vi "LESSON2_VIDEO8_CREATING_FIRST_APPLICATION.vi"() -> ()   [LabVIEW 2022 SP3]
panel:
  in  "Stop Button":bool
  out "Temperature Chart":dbl(graph)
  in  "Delay Multiplier":dbl(knob) scale=0.0..1.0
  in  "Number of Measurements":dbl
  # "This front panel shows chart numeric control and delay multiplier knob"
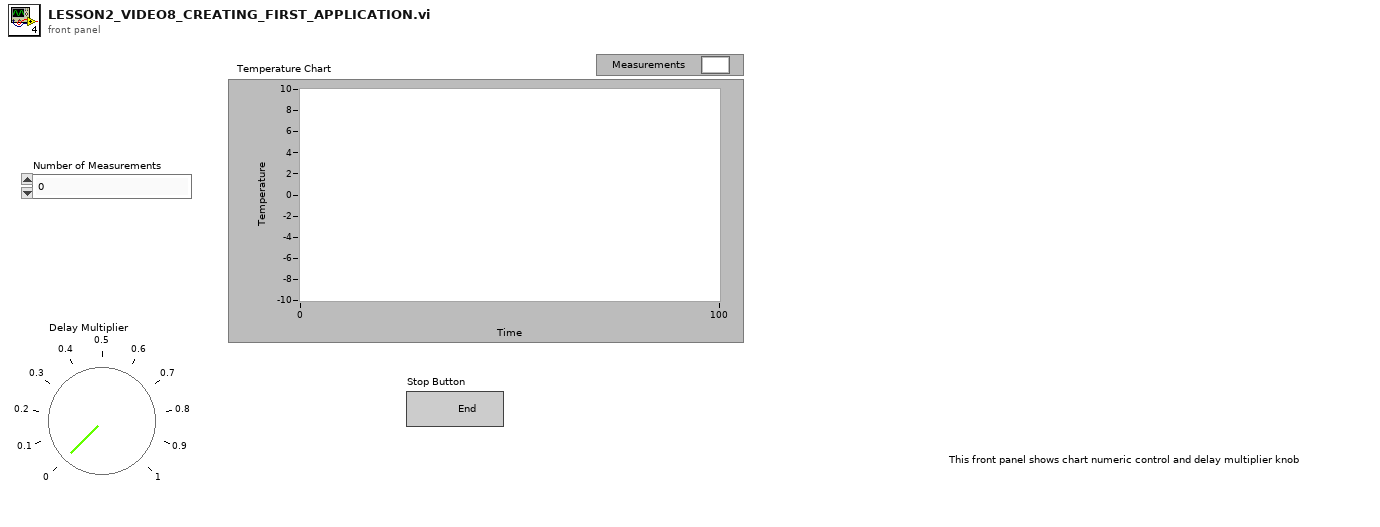
[diagram p1: front panel]
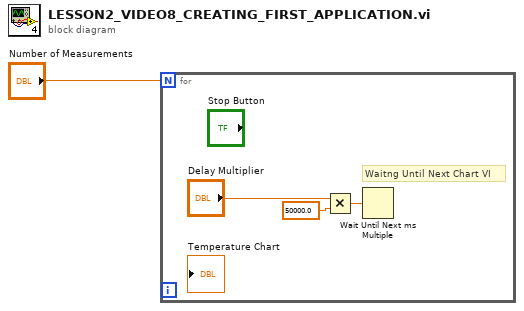
[diagram p0: block diagram]
diagram:
  n1 = for {
    N: "Number of Measurements" -> [_]
    # "Waitng Until Next Chart VI"
    n2 = Multiply(x="Delay Multiplier", y=50000.0) -> (x*y=w2:dbl)
    n3 = Wait Until Next ms Multiple(millisecond multiple=w2) -> ()  [unwired: 1 out]
  }
